vi "Calculate COB-ID from EBNF.vi"(8 "error in":errorcluster, 10 "ENBF":string, 11 "Transmit PDO in":refnum<class "PDO Communication Parameter.lvclass">) -> (0 "error out":errorcluster, 2 "COB-ID":u32, 3 "Transmit PDO out":refnum<class "PDO Communication Parameter.lvclass">)   [LabVIEW 2019, in "PDO Grid.lvlib" / "PDO Communication Parameter.lvclass"]
doc: "Parses Node-ID from Extended Backus-Naur formula in PDO communication sub-index 1 defaultvalue"
uses:
  PDO Communication Parameter.lvclass
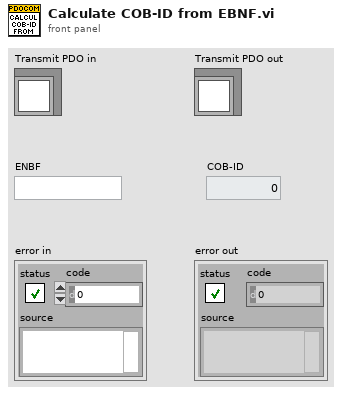
[diagram p1: front panel]
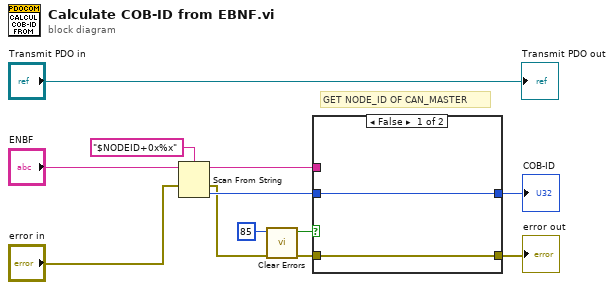
[diagram p0: block diagram]
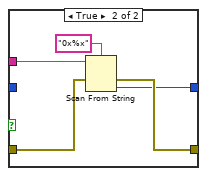
[diagram p2: hidden frame]
diagram:
  # "GET NODE_ID OF CAN_MASTER"
  n1 = Scan From String(format string="$NODEID+0x%x", input string="ENBF", error in="error in") -> (remaining string=w8:string, error out=w4:errorcluster, output 1=w7:u32)  [unwired: 2 in, 1 out]
  n2 = call <vilib>:"Clear Errors.vi"("error in (no error)"=w4, "specific error code to clear (0: all)"=85) -> ("error out"=w1:errorcluster, "specific error cleared?"=w2:bool)  [unwired: 4 in]
  n3 = case shown="False" w2 {
    tunnel: w8 -> [_ w19]
    tunnel: w7 -> [w14 _]
    tunnel: [w14 w15] -> w6
    tunnel: [w13 w16] -> w5
    tunnel: w1 -> [w13 w17]
    frame False {
    }
    frame True {
      n4 = Scan From String(format string="0x%x", input string=w19, error in=w17) -> (error out=w16:errorcluster, output 1=w15:u32)  [unwired: 2 in, 2 out]
    }
  }
  "error out" <- w5
  "COB-ID" <- w6
  "Transmit PDO out" <- "Transmit PDO in"
